vi "iRobot Navigation Target.vi"() -> ()   [LabVIEW 2013]
uses:
  iRobot Sensors.ctl
  iRobot Navigation State Machine.lvsc/StatechartState.ctl
  iRobot Navigation State Machine.lvsc/State.ctl
  Accel Filtered.ctl
  iRobot Navigation State Machine.lvsc/Inputs.ctl
  Accelerometer.ctl
  iRobot/Sensor/Sensor Group 6.ctl
  iRobot/Sensor/Bumps + Wheel Drops.ctl
  iRobot/Sensor/Low-Side Driver + Wheel Overcurrent.ctl
  iRobot/Sensor/Buttons.ctl
  iRobot/Sensor/Charging State.ctl
  iRobot/Sensor/Cargo Bay Digital Inputs.ctl
  iRobot/Sensor/Charging Sources Available.ctl
  iRobot/Sensor/OI Mode.ctl
  iRobot Navigation State Machine.lvsc/CompanionDiagram.vi/66/SC Main.vi
  iRobot Navigation State Machine.lvsc/CompanionDiagram.vi/66/Upd State.vi
  iRobot Navigation State Machine.lvsc/CompanionDiagram.vi/66/Trans Graph0.vi
  iRobot Navigation State Machine.lvsc/CompanionDiagram.vi/66/EnterGraphCore.vi
  <vilib>/myRIO/Common/Instrument Driver Framework/myRIO v1.0/UART/vis/myRIO v1.0 Close UART.vi
  iRobot Navigation State Machine.lvsc/CompanionDiagram.vi/66/Trans Graph1.vi
  iRobot Navigation State Machine.lvsc/CompanionDiagram.vi/66/Trans Graph2.vi
  iRobot Navigation State Machine.lvsc/CompanionDiagram.vi/66/Trans Graph3.vi
  <vilib>/Analysis/coordinate.llb/Wrap Angle.vi
  <vilib>/Analysis/coordinate.llb/Wrap Angle (scalar).vi
  <vilib>/FPGAPlugInAG/myRIO-1900/niLvFpga_Open_myRIO-1900.vi
  <vilib>/rvi/interface/common/dynamic/niFpgaDynamicAddResources.vi
  <vilib>/myRIO/Common/Instrument Driver Framework/Utilities/vis/FPGA Ref Manager.vi
  <vilib>/Utility/error.llb/Error Cluster From Error Code.vi
  iRobot Navigation State Machine.lvsc/CompanionDiagram.vi
  Hamming Distance.vi
  Create Message.vi
  Process Message.vi
  Select.vi
  Wheel Speed Filter.vi
  <vilib>/myRIO/Common/Instrument Driver Framework/myRIO v1.0/myRIO v1.0 Reset FPGA.vi
  <vilib>/FPGAPlugInAG/Dynamic/niLvFpga_Close_Dynamic.vi
  iRobot Navigation State Machine.lvsc/Trigger.ctl
  <vilib>/rvi/interface/nirviOpenFPGA/nirviOpenFPGA.xnode
  LED Matrix/FPGA Bitfiles/LEDMatrix4_FPGATarget_myRIO-1900Custom_r1aLzQW2H5E.lvbitx
  <vilib>/Statechart/Infrastructure/RTStatechart/RunTime SCN.xnode
  iRobot Navigation State Machine.lvsc/Outputs.ctl
  iRobot Navigation State Machine.lvsc
  <vilib>/rvi/interface/nirviCloseFPGA/nirviCloseFPGA.xnode
  <vilib>/myRIO/Instrument Drivers/Utilities/Utilities.lvlib
panel:
  out "Max Filtered Accelerometer":T1 {"All Mag" format="%_3f"; "Vert Mag" format="%_3f"; "x axis (g)" format="%_3f"; "y axis (g)" format="%_3f"; "z axis (g)" format="%_3f"; "Horiz Mag" format="%_3f"}
  out "Max Filtered Accelerometer Delta":T1 {"All Mag" format="%_3f"; "Vert Mag" format="%_3f"; "x axis (g)" format="%_3f"; "y axis (g)" format="%_3f"; "z axis (g)" format="%_3f"; "Horiz Mag" format="%_3f"}
  in  "Reset Accel Max":bool
  in  "Reset Delta Max":bool
  out "Hamming Dist":u32
  out "LED Matrix":picture
  in  "Tab Control":T2(tab)
  out "iRobot Sensors (graphical)":T3 {"Right Wheel (mm/s)" scale=-500.0..500.0; "Left Wheel (mm/s)" scale=-500.0..500.0}
  out "Active States":T5
  out "error out":errorcluster
  in  "Wheel Speed (mm/s)":i16(slide)=100 scale=0.0..500.0
  in  "accel smoothing (0-1)":dbl=1.0
  in  "filter factor (0-1)":dbl=0.02
  in  "stop":bool
  out "Target Running":bool
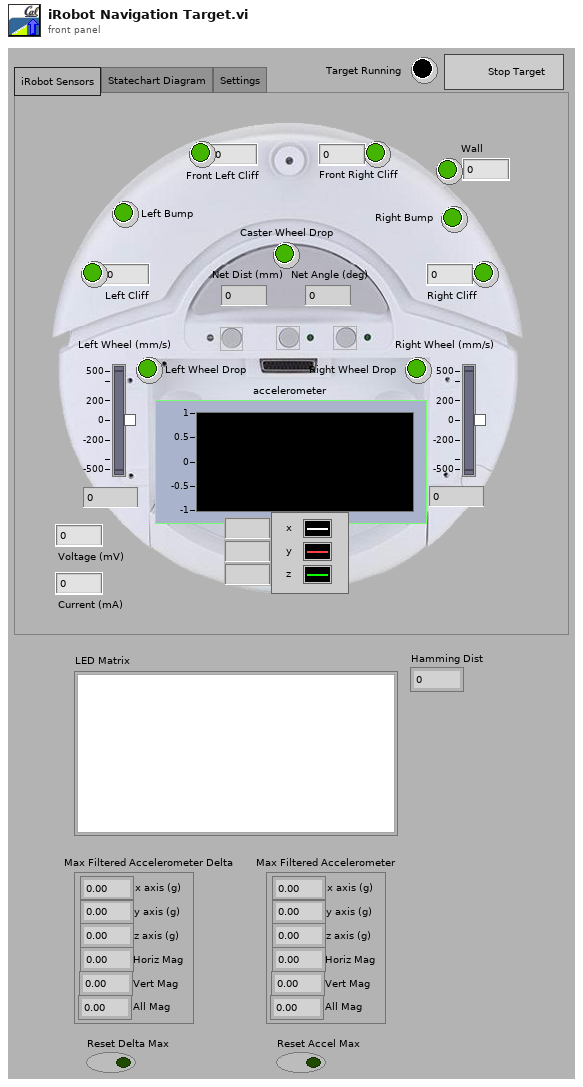
[diagram p1: front panel]
types:
  T1 = typedef "Accel Filtered.ctl" = cluster{"x axis (g)":dbl, "y axis (g)":dbl, "z axis (g)":dbl, "Horiz Mag":dbl, "Vert Mag":dbl, "All Mag":dbl}
  T2 = enum32{"iRobot Sensors", "Statechart Diagram", "Settings"}
  T3 = typedef "iRobot Sensors.ctl" = cluster{"Caster Wheel Drop":bool, "Left Wheel Drop":bool, "Right Wheel Drop":bool, "Left Bump":bool, "Right Bump":bool, "Left Cliff":bool, "Front Left Cliff":bool, "Front Right Cliff":bool, "Right Cliff":bool, "Wall":bool, "Net Dist (mm)":i32, "Net Angle (deg)":i32, "Wall":u16, "Left Cliff":u16, "Front Left Cliff":u16, "Front Right Cliff":u16, "Right Cliff":u16, "Left Wheel (mm/s)":i16, "Right Wheel (mm/s)":i16, "accelerometer":T4, "Voltage (mV)":dbl, "Current (mA)":dbl}
  T4 = typedef "Accelerometer.ctl" = cluster{"x axis (g)":dbl, "y axis (g)":dbl, "z axis (g)":dbl}
  T5 = typedef "iRobot Navigation State Machine.lvsc/StatechartState.ctl" = T6[]
  T6 = typedef "iRobot Navigation State Machine.lvsc/State.ctl" = enum16{"NI.SC.Initial", "NI.SC.History", "NI.SC.ShallowHistory", "NI.SC.Terminal", "End", "Running", "Start", "Running\\NI.SC.UnnamedRegion 0\\Genetic Algorithm", "Running\\NI.SC.UnnamedRegion 0\\Detect Collision", "Running\\NI.SC.UnnamedRegion 0\\Move Around", "Running\\NI.SC.UnnamedRegion 0\\Update LED", "Running\\NI.SC.UnnamedRegion 0\\Genetic Algorithm\\NI.SC.UnnamedRegion 0\\Determine\nNew Parent", "Running\\NI.SC.UnnamedRegion 0\\Genetic Algorithm\\NI.SC.UnnamedRegion 0\\Transfer Runnersup", "Running\\NI.SC.UnnamedRegion 0\\Genetic Algorithm\\NI.SC.UnnamedRegion 0\\Select Best", "Running\\NI.SC.UnnamedRegion 0\\Genetic Algorithm\\NI.SC.UnnamedRegion 0\\Get Other Parent", "Running\\NI.SC.UnnamedRegion 0\\Move Around\\NI.SC.UnnamedRegion 0\\Back Up", "Running\\NI.SC.UnnamedRegion 0\\Move Around\\NI.SC.UnnamedRegion 0\\Turn", "Running\\NI.SC.UnnamedRegion 0\\Move Around\\NI.SC.UnnamedRegion 0\\Drive"}
  T7 = typedef "iRobot UART Port Type.ctl" = refnum<visa-resource-name>
  T8 = typedef "iRobot Navigation State Machine.lvsc/Inputs.ctl" = cluster{"net distance (mm)":i32, "net angle (deg)":i32, "Max Wheel Speed (mm/s)":i16, "accelerometer":T4, "iRobot Sensors":T9, "Is Simulator?":bool, "Filtered Accelerometer":T1, "Filtered Accel Delta":T1}
  T9 = typedef "Sensor Group 6.ctl" = cluster{"Bumps + Wheel Drops":T10, "Wall":bool, "Cliff Left":bool, "Cliff Front Left":bool, "Cliff Front Right":bool, "Cliff Right":bool, "Virtual Wall":bool, "Low-Side Driver + Wheel Overcurrent":T11, "Infrared":u8, "Buttons":T12, "Distance (mm)":i32, "Angle (deg)":i32, "Charging State":T13, "Voltage (mV)":u16, "Current (mA)":i16, "Battery Temperature (deg C)":i8, "Battery Charge (mAh)":u16, "Battery Capacity (mAh)":u16, "Wall Signal (0-4095)":u16, "Cliff Left Signal (0-4095)":u16, "Cliff Front Left Signal (0-4095)":u16, "Cliff Front Right Signal (0-4095)":u16, "Cliff Right Signal (0-4095)":u16, "Cargo Bay Digital Inputs":T14, "Cargo Bay Analog Signal (0-1023)":u16, "Charging Sources Available":T15, "OI Mode":T16, "Song Number":u8, "Song Playing":bool, "Number of Stream Packets":u8, "Requested Velocity (mm/s)":i16, "Requested Radius (mm)":i16, "Requested Right Wheel Velocity (mm/s)":i16, "Requested Left Wheel Velocity (mm/s)":i16}
  T10 = typedef "Bumps + Wheel Drops.ctl" = cluster{"Wheeldrop Caster":bool, "Wheeldrop Left":bool, "Wheeldrop Right":bool, "Bump Left":bool, "Bump Right":bool}
  T11 = typedef "Low-Side Driver + Wheel Overcurrent.ctl" = cluster{"Low-Side Driver 0":bool, "Low-Side Driver 1":bool, "Low-Side Driver 2":bool, "Left Wheel":bool, "Right Wheel":bool}
  T12 = typedef "Buttons.ctl" = cluster{"Advance":bool, "Play":bool}
  T13 = typedef "Charging State.ctl" = enum16{"Not Charging", "Reconditioning Charging", "Full Charging", "Trickle Charging", "Waiting", "Charging Fault Condition"}
  T14 = typedef "Cargo Bay Digital Inputs.ctl" = cluster{"Digital Input 0":bool, "Digital Input 1":bool, "Digital Input 2":bool, "Digital Input 3":bool, "Device Detect":bool}
  T15 = typedef "Charging Sources Available.ctl" = cluster{"Internal Charger":bool, "Home Base":bool}
  T16 = typedef "OI Mode.ctl" = enum16{"Off", "Passive", "Safe", "Full"}
  T17 = typedef "iRobot Navigation State Machine.lvsc/Outputs.ctl" = cluster{"Left Wheel Speed (mm/s)":i16, "Right Wheel Speed (mm/s)":i16, "Parent":u8[], "Hamming Dist":u32, "Last Bytes Written":i32, "TCP Error":errorcluster}
  T18 = cluster{"[0]":dbl, "[1]":dbl, "[2]":dbl, "[3]":dbl, "[4]":dbl, "[5]":dbl}
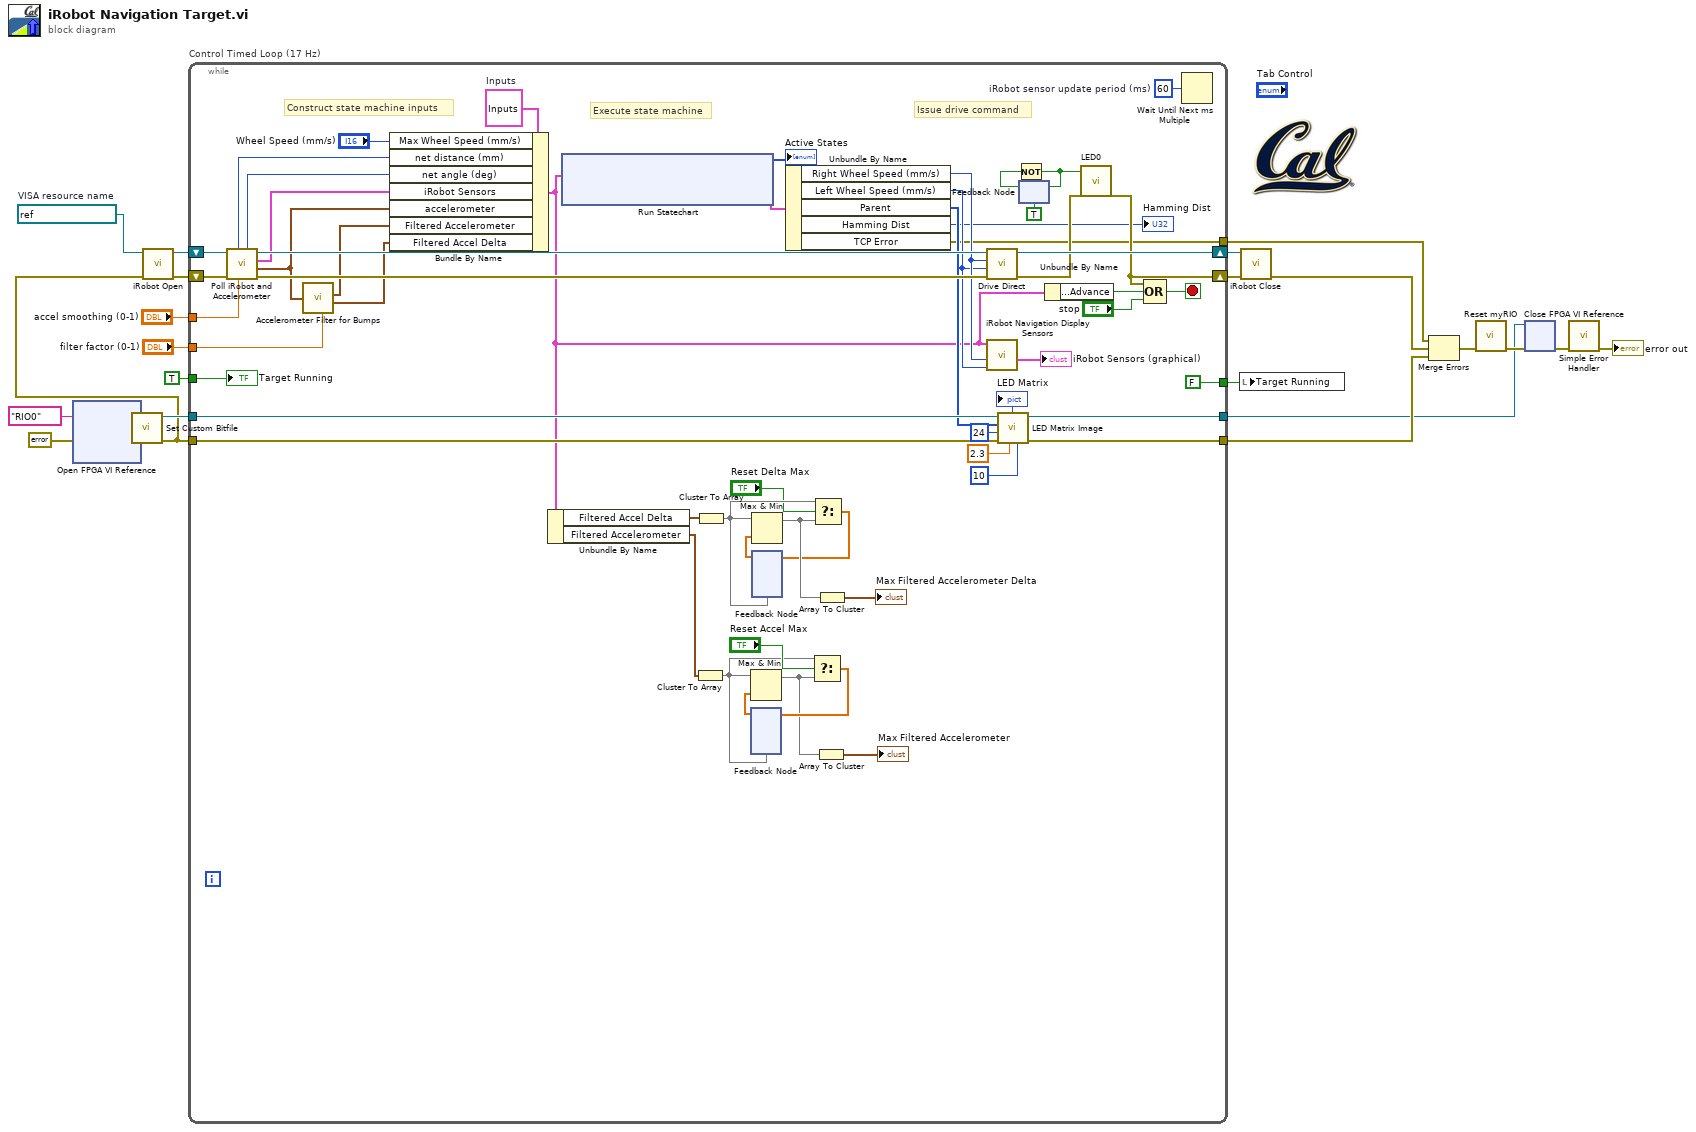
[diagram p0: block diagram]
diagram:
  w17 = refnum<visa-resource-name> "ASRL1::INSTR"  # VISA resource name
  n1 = xnode "Open FPGA VI Reference"("error in"=errorcluster {"status"=FALSE, "code"=0, "source"=""}, "resource name"=tag "RIO0") -> ("FPGA VI Reference Out"=w14:refnum<k20>, "error out"=w15:errorcluster)
  n2 = call <vilib>:"Set Custom Bitfile.vi"("error in (no error)"=w15, "Customized FPGA Reference in"=w14) -> ("error out"=w10:errorcluster, "Customized FPGA Reference out"=w12:refnum<k20>)  [unwired: 8 in]
  n3 = call "iRobot Open.vi"("error in (no error)"=w10, "UART port in"=w17) -> ("error out"=w22:errorcluster, "UART port out"=w21:T7)  [unwired: 8 in]
  n4 = while "Control Timed Loop (17 Hz)" {
    shift-right: [w80] -> w23
    shift-left: w21 -> [w75]
    shift-right: [w62] -> w18
    shift-left: w22 -> [w74]
    tunnel: TRUE ("stop") -> [w68]
    tunnel: [FALSE ("stop")] -> w19
    tunnel: "accel smoothing (0-1)" -> [w55]
    tunnel: w12 -> [w53]
    tunnel: w10 -> [w52]
    tunnel: [w46] -> w2
    tunnel: [w45] -> w6
    tunnel: [w43] -> w5
    tunnel: "filter factor (0-1)" -> [w39]
    stop <- w79 stop-if-true
    w54 = u32 60  # iRobot sensor update period (ms)
    w77 = T8 {"net distance (mm)"=0, "net angle (deg)"=0, "Max Wheel Speed (mm/s)"=0, "accelerometer"={"x axis (g)"=0.0, "y axis (g)"=0.0, "z axis (g)"=0.0}, "iRobot Sensors"={"Bumps + Wheel Drops"={"Wheeldrop Caster"=FALSE, "Wheeldrop Left"=FALSE, "Wheeldrop Right"=FALSE, "Bump Left"=FALSE, "Bump Right"=FALSE}, "Wall"=FALSE, "Cliff Left"=FALSE, "Cliff Front Left"=FALSE, "Cliff Front Right"=FALSE, "Cliff Right"=FALSE, "Virtual Wall"=FALSE, "Low-Side Driver + Wheel Overcurrent"={"Low-Side Driver 0"=FALSE, "Low-Side Driver 1"=FALSE, "Low-Side Driver 2"=FALSE, "Left Wheel"=FALSE, "Right Wheel"=FALSE}, "Infrared"=255, "Buttons"={"Advance"=FALSE, "Play"=FALSE}, "Distance (mm)"=0, "Angle (deg)"=0, "Charging State"=enum."Not Charging", "Voltage (mV)"=0, "Current (mA)"=0, "Battery Temperature (deg C)"=0, "Battery Charge (mAh)"=0, "Battery Capacity (mAh)"=0, "Wall Signal (0-4095)"=0, "Cliff Left Signal (0-4095)"=0, "Cliff Front Left Signal (0-4095)"=0, "Cliff Front Right Signal (0-4095)"=0, "Cliff Right Signal (0-4095)"=0, "Cargo Bay Digital Inputs"={"Digital Input 0"=FALSE, "Digital Input 1"=FALSE, "Digital Input 2"=FALSE, "Digital Input 3"=FALSE, "Device Detect"=FALSE}, "Cargo Bay Analog Signal (0-1023)"=0, "Charging Sources Available"={"Internal Charger"=FALSE, "Home Base"=FALSE}, "OI Mode"=enum."Off", "Song Number"=0, "Song Playing"=FALSE, "Number of Stream Packets"=0, "Requested Velocity (mm/s)"=0, "Requested Radius (mm)"=0, "Requested Right Wheel Velocity (mm/s)"=0, "Requested Left Wheel Velocity (mm/s)"=0}, "Is Simulator?"=FALSE, "Filtered Accelerometer"={"x axis (g)"=0.0, "y axis (g)"=0.0, "z axis (g)"=0.0, "Horiz Mag"=0.0, "Vert Mag"=0.0, "All Mag"=0.0}, "Filtered Accel Delta"={"x axis (g)"=0.0, "y axis (g)"=0.0, "z axis (g)"=0.0, "Horiz Mag"=0.0, "Vert Mag"=0.0, "All Mag"=0.0}}  # Inputs
    # "Issue drive command"
    # "Execute state machine"
    # "Construct state machine inputs"
    n5 = call "Poll iRobot and Accelerometer.vi"("accel smoothing (0-1)"=w55, "error in"=w74, "UART port in"=w75) -> ("error out"=w73:errorcluster, "Acceleration (g)"=w42:T4, "iRobot SensorGroup6"=w61:T9, "UART port out"=w72:T7, "net angle (deg)"=w70:i32, "net distance (mm)"=w71:i32)  [unwired: 3 in]
    n6 = call "Accelerometer Filter for Bumps.vi"("filter factor (0-1)"=w39, "accelerometer (g)"=w42) -> ("filtered out"=w41:T1, "abs delta"=w40:T1)  [unwired: 4 in]
    n7 = Bundle By Name(cluster=w77, "Max Wheel Speed (mm/s)"="Wheel Speed (mm/s)", "net distance (mm)"=w71, "net angle (deg)"=w70, "iRobot Sensors"=w61, "accelerometer"=w42, "Filtered Accelerometer"=w41, "Filtered Accel Delta"=w40) -> (w26:T8)
    n8 = Unbundle By Name(w26) -> ("Filtered Accel Delta"=w27:T1, "Filtered Accelerometer"=w28:T1)
    n9 = xnode "Run Statechart"("Inputs"=w26) -> ("Outputs"=w78:T17, "Active States"=→"Active States":T5)  [unwired: 2 in, 1 out]
    n10 = Cluster To Array(cluster=w28) -> (array=w31:dbl[])
    n11 = Cluster To Array(cluster=w27) -> (array=w36:dbl[])
    n12 = feedback #1(w31) -> (w32:dbl[])
    n13 = Max & Min(x=w31, y=w32) -> (max(x,y)=w29:dbl[])  [unwired: 1 out]
    n14 = feedback #2(w36) -> (w35:dbl[])
    n15 = Max & Min(x=w36, y=w35) -> (max(x,y)=w38:dbl[])  [unwired: 1 out]
    n16 = Unbundle By Name(w78) -> ("Right Wheel Speed (mm/s)"=w59:i16, "Left Wheel Speed (mm/s)"=w58:i16, "Parent"=w51:u8[], "Hamming Dist"=→"Hamming Dist":u32, "TCP Error"=w43:errorcluster)
    n17 = Select(t=w31, s="Reset Accel Max", f=w29) -> (s? t:f=w30:dbl[])
    n18 = feedback-in #1(w30) -> ()
    n19 = Select(t=w36, s="Reset Delta Max", f=w38) -> (s? t:f=w37:dbl[])
    n20 = feedback-in #2(w37) -> ()
    n21 = Array To Cluster(array=w29) -> (cluster=→"Max Filtered Accelerometer":T18)
    n22 = Array To Cluster(array=w38) -> (cluster=→"Max Filtered Accelerometer Delta":T18)
    n23 = call "Drive Direct.vi"("error in"=w73, "Left Wheel Velocity (mm/s)"=w58, "Right Wheel Velocity (mm/s)"=w59, "UART port in"=w72) -> ("error out"=w63:errorcluster, "UART port out"=w80:T7)  [unwired: 6 in]
    n24 = call "iRobot Navigation Display Sensors.vi"("Left Wheel (mm/s)"=w58, "Right Wheel (mm/s)"=w59, "Statechart Inputs"=w26) -> ("iRobot Sensors (graphical)"=→"iRobot Sensors (graphical)":T3)  [unwired: 6 in]
    n25 = call "LED Matrix Image.vi"("Brightness"=u8 10, "Factor"=2.3, "error in (no error)"=w52, "image depth"=24, "image"=w51, "Refnum in"=w53) -> ("error out"=w45:errorcluster, "Refnum out"=w46:refnum<k20>, "LED Matrix"=→"LED Matrix":picture)  [unwired: 3 in]
    n26 = feedback #3(TRUE) -> (w64:bool)
    n27 = Not(x=w64) -> (.not. x?=w65:bool)
    n28 = feedback-in #3(w65) -> ()
    n29 = Unbundle By Name(w26) -> ("iRobot Sensors.Buttons.Advance"=w56:bool)
    n30 = call "LED0"("LED0"=w65, "error in (no error)"=w63) -> ("error out"=w62:errorcluster)  [unwired: 25 in]
    n31 = Compound Arithmetic op=OR(w62, w56, "stop") -> (w79:bool)
    n32 = Wait Until Next ms Multiple(millisecond multiple=w54) -> ()  [unwired: 1 out]
    "Target Running" <- w68
  }
  n33 = local write "Target Running"(w19) -> ()
  n34 = call "iRobot Close.vi"("error in"=w18, "UART port in"=w23) -> ("error out"=w7:errorcluster)  [unwired: 9 in]
  n35 = Merge Errors(w5, w7, w6) -> (w8:errorcluster)
  n36 = call <vilib>:"Reset myRIO.vi"("error in (no error)"=w8) -> ("error out"=w4:errorcluster)  [unwired: 10 in]
  n37 = xnode "Close FPGA VI Reference"("FPGA VI Reference In"=w2, "error in"=w4) -> ("error out"=w3:errorcluster)
  n38 = call <vilib>:"Simple Error Handler.vi"("error in (no error)"=w3) -> ("error out"=→"error out":errorcluster)  [unwired: 4 in, 4 out]
